vi "Vision Processing.vi"(4 "error in (no error)":errorcluster, 7 "Image Size":T4=enum."320x240") -> ()   [LabVIEW 2020]
doc: "This VI runs in parallel to other tasks. It gets images from the camera, processes them for color or shape and use that information to affect robot behavior."
uses:
  Robot Global Data.vi
  <vilib>/Rock Robotics/WPI/Camera/WPI_CameraWhite Balance Values.ctl
  <vilib>/Rock Robotics/WPI/Camera/WPI_CameraExposure Values.ctl
  <vilib>/Rock Robotics/WPI/Camera/WPI_CameraFrameRate.ctl
  <vilib>/Rock Robotics/Network Tables/NT Read Number.vi
  <vilib>/Rock Robotics/Network Tables/NT Write Boolean.vi
  <vilib>/Rock Robotics/Network Tables/NT Write Number.vi
  <vilib>/Rock Robotics/Network Tables/NT Read Boolean.vi
  <vilib>/Rock Robotics/WPI/Camera/WPI_CameraImageSize.ctl
panel:
  in  "Std Devs":cluster{"Hue":dbl, "Sat":dbl, "Val":dbl}={"Hue"=4.0, "Sat"=6.0, "Val"=4.0}
  in  "Color Components":T1={"Hue"={243.23333311080933, 20.233333110809326}, "Sat"={125.60287475585938, 242.93045043945312}, "Val"={83.88507843017578, 225.38158416748047}} {"Val" scale=0.0..255.0; "Sat" scale=0.0..255.0; "Hue" scale=0.0..255.0 scale format="%#_3g"}
  out "Fitted Mask":T2(plugin-control)
  in  "Targets":i32=3
  in  "Score Cutoff":dbl(slide)=70.58823529411765 scale=0.0..100.0
  out "Ranked Objects":T3(array[cluster]) {"Score" format="%#.1g"}
  in  "Annotations":enum16{"None", "Good", "All"}(ring)=enum."Good"
  in  "Area Size Limit %":dbl=0.4 format="%#_13g"
  out "Initial Mask":T2(plugin-control)
  out "Image":T2(plugin-control)
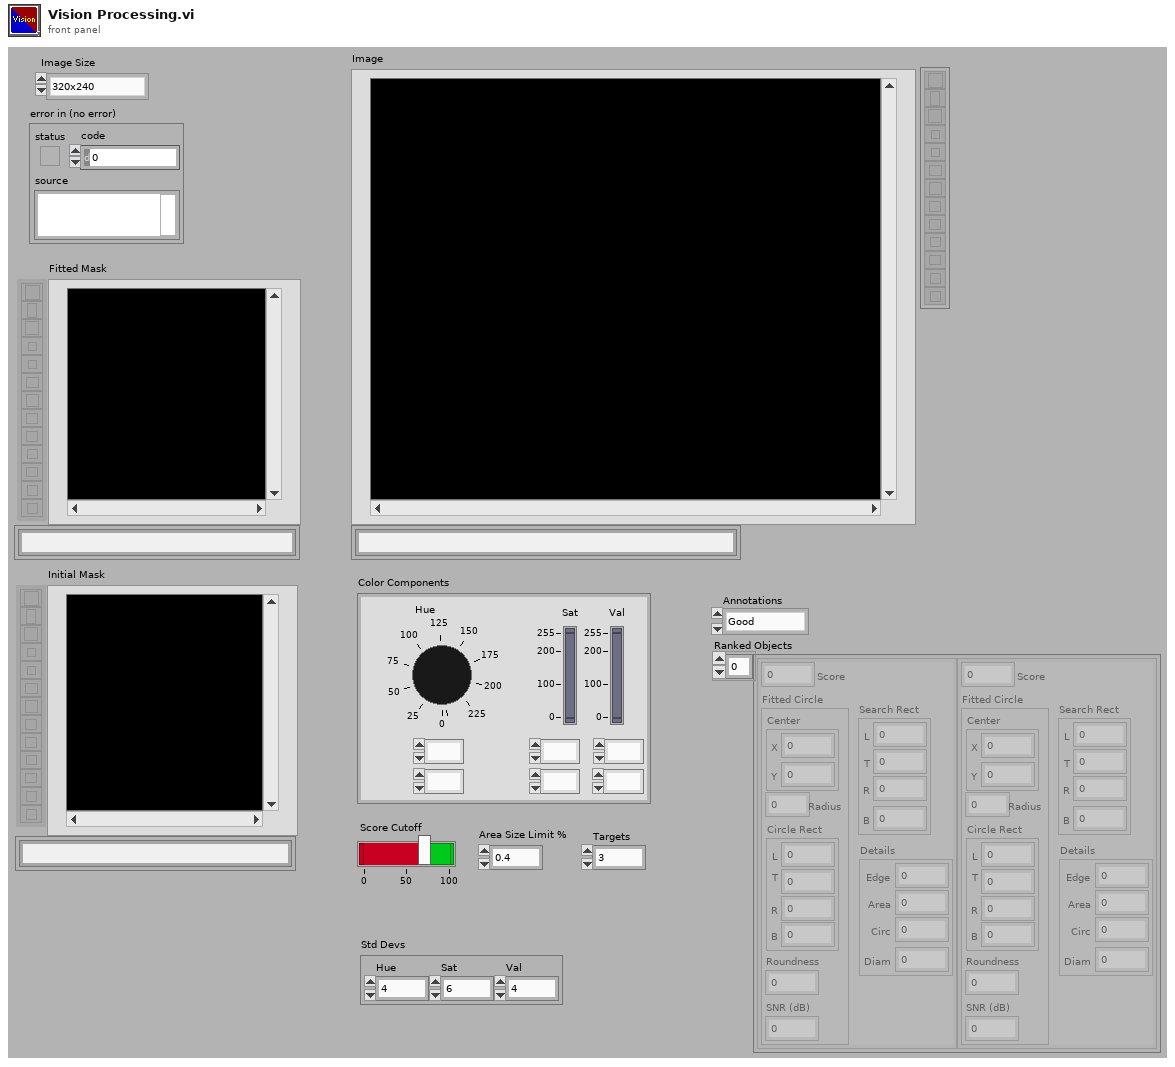
[diagram p1: front panel]
types:
  T1 = cluster{"Hue":cluster{dbl, dbl}, "Sat":cluster{dbl, dbl}, "Val":cluster{dbl, dbl}}
  T2 = typedef "IMAQ Image.ctl" = refnum<image>
  T3 = cluster{"Score":sgl, "Fitted Circle":cluster{"Center":cluster{"X":sgl, "Y":sgl}, "Radius":dbl, "Circle Rect":cluster{"L":sgl, "T":sgl, "R":sgl, "B":sgl}, "Roundness":dbl, "SNR (dB)":dbl}, "Search Rect":cluster{"L":sgl, "T":sgl, "R":sgl, "B":sgl}, "Details":cluster{"Edge":sgl, "Area":sgl, "Circ":sgl, "Diam":sgl}}[]
  T4 = typedef "WPI_CameraImageSize.ctl" = enum16{"640x480", "320x240", "160x120", "Custom"}
  T5 = typedef "WPI_CameraFrameRate.ctl" = u32
  T6 = typedef "WPI_CameraExposure Values.ctl" = enum16{"Auto", "Flicker-free 50 Hz", "Flicker-free 60 Hz", "Hold current", "Custom"}
  T7 = typedef "WPI_CameraWhite Balance Values.ctl" = enum16{"Auto", "Fixed indoor", "Fixed outdoor 1", "Fixed outdoor 2", "Fixed fluorescent 1", "Fixed fluorescent 2", "Hold current", "Custom"}
  T8 = typedef "Image Type" = u32
  T9 = typedef "WPI_CameraDevRef.ctl" = cluster{"Camera Address":string, "CameraStatus":errorcluster}
  T10 = typedef "WPI_DriverStationAllianceInfo.ctl" = enum16{"Red", "Blue", "Invalid"}
  T11 = cluster{cluster{"Numeric":dbl, "Numeric":dbl}, cluster{"Numeric":dbl, "Numeric":dbl}, cluster{"Numeric":dbl, "Numeric":dbl}}
  T12 = cluster{"Hue":cluster{"Numeric":dbl, "Numeric":dbl}, "Sat":cluster{"Numeric":dbl, "Numeric":dbl}, "Val":cluster{"Numeric":dbl, "Numeric":dbl}}
  T13 = cluster{"Circle Found":bool, "Fitted Circle":cluster{"Center":cluster{"X":sgl, "Y":sgl}, "Radius":dbl, "Center":cluster{"X":sgl, "Y":sgl}, "Radius":dbl, "Roundness":dbl, "Strength":dbl, "SNR (dB)":dbl}, "Array":dbl[], "Sorted Data":dbl[][]}[]
  T14 = cluster{cluster{dbl, dbl}, cluster{dbl, dbl}, cluster{dbl, dbl}}
  T15 = cluster{"Score":dbl, "Fitted Circle":cluster{"Center (Pixels)":cluster{"X":sgl, "Y":sgl}, "Radius (Pixels)":dbl, "Circle Rect":cluster{"Left":sgl, "Top":sgl, "Right":sgl, "Bottom":sgl}, "Roundness (RW)":dbl, "Average SNR (dB)":dbl}, "Search Rect":cluster{"Left":sgl, "Top":sgl, "Right":sgl, "Bottom":sgl}, "Details":cluster{"Edges":sgl, "Circ/Rect":sgl, "Diam/Diam":sgl, "Circularity":sgl}}[]
  T16 = cluster{"Object Info[0]":cluster{"Score":dbl, "Fitted Circle":cluster{"Center (Pixels)":cluster{"X":sgl, "Y":sgl}, "Radius (Pixels)":dbl, "Circle Rect":cluster{"Left":sgl, "Top":sgl, "Right":sgl, "Bottom":sgl}, "Roundness (RW)":dbl, "Average SNR (dB)":dbl}, "Search Rect":cluster{"Left":sgl, "Top":sgl, "Right":sgl, "Bottom":sgl}, "Details":cluster{"Edges":sgl, "Circ/Rect":sgl, "Diam/Diam":sgl, "Circularity":sgl}}, "Object Info[1]":cluster{"Score":dbl, "Fitted Circle":cluster{"Center (Pixels)":cluster{"X":sgl, "Y":sgl}, "Radius (Pixels)":dbl, "Circle Rect":cluster{"Left":sgl, "Top":sgl, "Right":sgl, "Bottom":sgl}, "Roundness (RW)":dbl, "Average SNR (dB)":dbl}, "Search Rect":cluster{"Left":sgl, "Top":sgl, "Right":sgl, "Bottom":sgl}, "Details":cluster{"Edges":sgl, "Circ/Rect":sgl, "Diam/Diam":sgl, "Circularity":sgl}}, "Object Info[2]":cluster{"Score":dbl, "Fitted Circle":cluster{"Center (Pixels)":cluster{"X":sgl, "Y":sgl}, "Radius (Pixels)":dbl, "Circle Rect":cluster{"Left":sgl, "Top":sgl, "Right":sgl, "Bottom":sgl}, "Roundness (RW)":dbl, "Average SNR (dB)":dbl}, "Search Rect":cluster{"Left":sgl, "Top":sgl, "Right":sgl, "Bottom":sgl}, "Details":cluster{"Edges":sgl, "Circ/Rect":sgl, "Diam/Diam":sgl, "Circularity":sgl}}, "Object Info[3]":cluster{"Score":dbl, "Fitted Circle":cluster{"Center (Pixels)":cluster{"X":sgl, "Y":sgl}, "Radius (Pixels)":dbl, "Circle Rect":cluster{"Left":sgl, "Top":sgl, "Right":sgl, "Bottom":sgl}, "Roundness (RW)":dbl, "Average SNR (dB)":dbl}, "Search Rect":cluster{"Left":sgl, "Top":sgl, "Right":sgl, "Bottom":sgl}, "Details":cluster{"Edges":sgl, "Circ/Rect":sgl, "Diam/Diam":sgl, "Circularity":sgl}}, "Object Info[4]":cluster{"Score":dbl, "Fitted Circle":cluster{"Center (Pixels)":cluster{"X":sgl, "Y":sgl}, "Radius (Pixels)":dbl, "Circle Rect":cluster{"Left":sgl, "Top":sgl, "Right":sgl, "Bottom":sgl}, "Roundness (RW)":dbl, "Average SNR (dB)":dbl}, "Search Rect":cluster{"Left":sgl, "Top":sgl, "Right":sgl, "Bottom":sgl}, "Details":cluster{"Edges":sgl, "Circ/Rect":sgl, "Diam/Diam":sgl, "Circularity":sgl}}, "Object Info[5]":cluster{"Score":dbl, "Fitted Circle":cluster{"Center (Pixels)":cluster{"X":sgl, "Y":sgl}, "Radius (Pixels)":dbl, "Circle Rect":cluster{"Left":sgl, "Top":sgl, "Right":sgl, "Bottom":sgl}, "Roundness (RW)":dbl, "Average SNR (dB)":dbl}, "Search Rect":cluster{"Left":sgl, "Top":sgl, "Right":sgl, "Bottom":sgl}, "Details":cluster{"Edges":sgl, "Circ/Rect":sgl, "Diam/Diam":sgl, "Circularity":sgl}}, "Object Info[6]":cluster{"Score":dbl, "Fitted Circle":cluster{"Center (Pixels)":cluster{"X":sgl, "Y":sgl}, "Radius (Pixels)":dbl, "Circle Rect":cluster{"Left":sgl, "Top":sgl, "Right":sgl, "Bottom":sgl}, "Roundness (RW)":dbl, "Average SNR (dB)":dbl}, "Search Rect":cluster{"Left":sgl, "Top":sgl, "Right":sgl, "Bottom":sgl}, "Details":cluster{"Edges":sgl, "Circ/Rect":sgl, "Diam/Diam":sgl, "Circularity":sgl}}, "Object Info[7]":cluster{"Score":dbl, "Fitted Circle":cluster{"Center (Pixels)":cluster{"X":sgl, "Y":sgl}, "Radius (Pixels)":dbl, "Circle Rect":cluster{"Left":sgl, "Top":sgl, "Right":sgl, "Bottom":sgl}, "Roundness (RW)":dbl, "Average SNR (dB)":dbl}, "Search Rect":cluster{"Left":sgl, "Top":sgl, "Right":sgl, "Bottom":sgl}, "Details":cluster{"Edges":sgl, "Circ/Rect":sgl, "Diam/Diam":sgl, "Circularity":sgl}}, "Object Info[8]":cluster{"Score":dbl, "Fitted Circle":cluster{"Center (Pixels)":cluster{"X":sgl, "Y":sgl}, "Radius (Pixels)":dbl, "Circle Rect":cluster{"Left":sgl, "Top":sgl, "Right":sgl, "Bottom":sgl}, "Roundness (RW)":dbl, "Average SNR (dB)":dbl}, "Search Rect":cluster{"Left":sgl, "Top":sgl, "Right":sgl, "Bottom":sgl}, "Details":cluster{"Edges":sgl, "Circ/Rect":sgl, "Diam/Diam":sgl, "Circularity":sgl}}}
  T17 = cluster{"Score":dbl, "Fitted Circle":cluster{"Center (Pixels)":cluster{"X":sgl, "Y":sgl}, "Radius (Pixels)":dbl, "Circle Rect":cluster{"Left":sgl, "Top":sgl, "Right":sgl, "Bottom":sgl}, "Roundness (RW)":dbl, "Average SNR (dB)":dbl}, "Search Rect":cluster{"Left":sgl, "Top":sgl, "Right":sgl, "Bottom":sgl}, "Details":cluster{"Edges":sgl, "Circ/Rect":sgl, "Diam/Diam":sgl, "Circularity":sgl}}
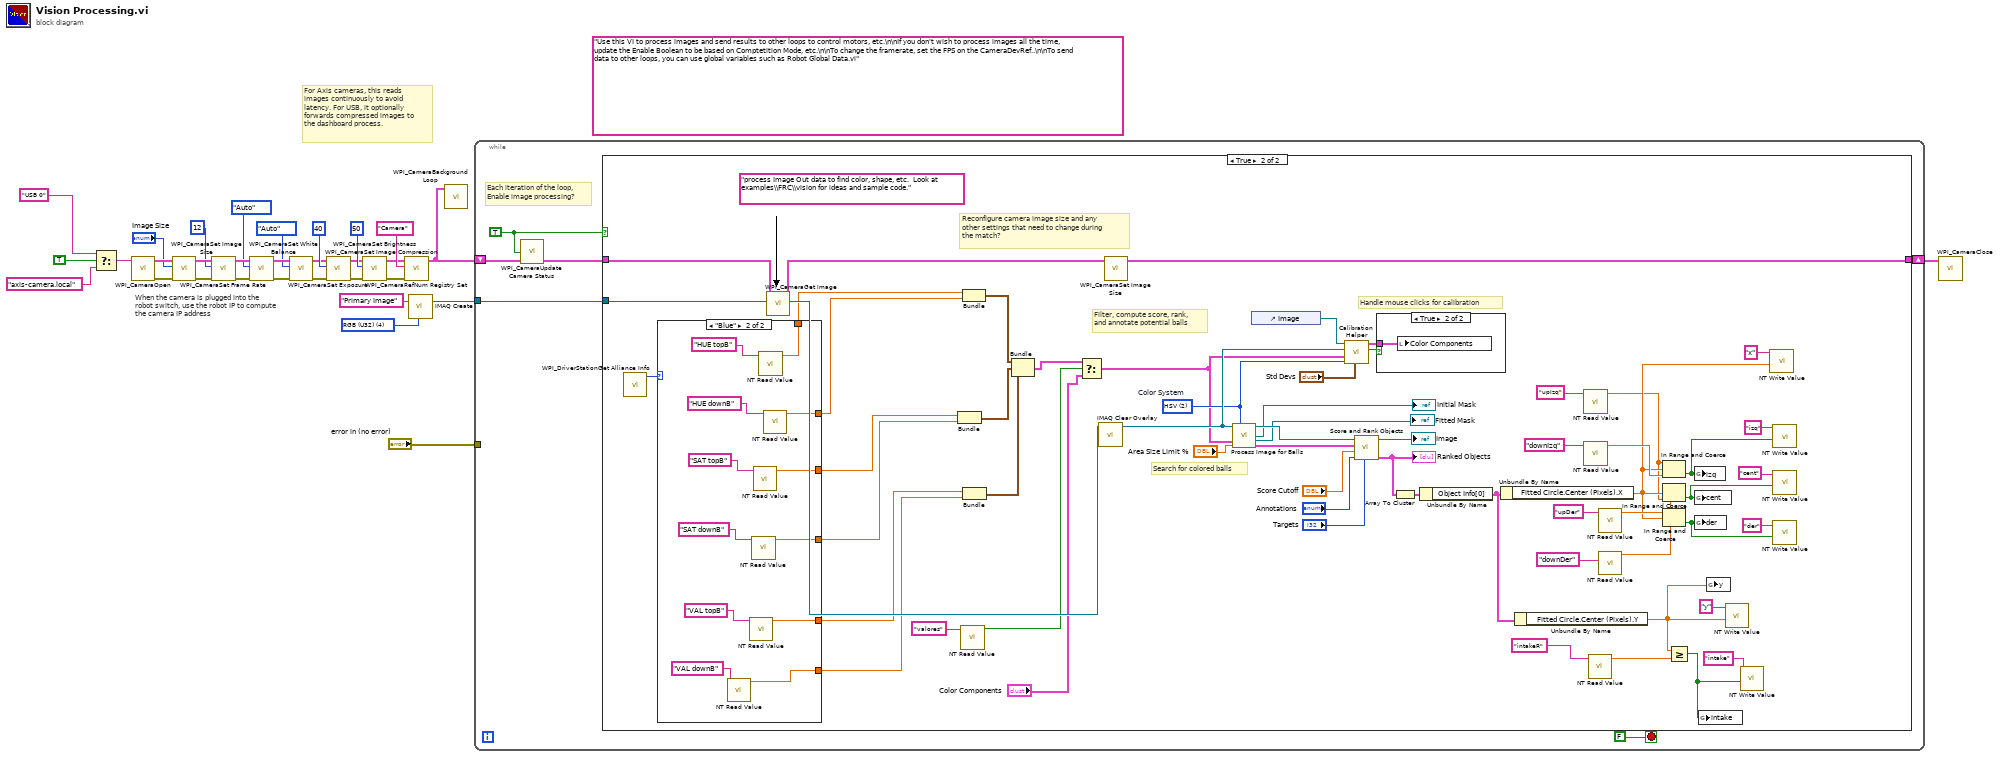
[diagram p0: block diagram]
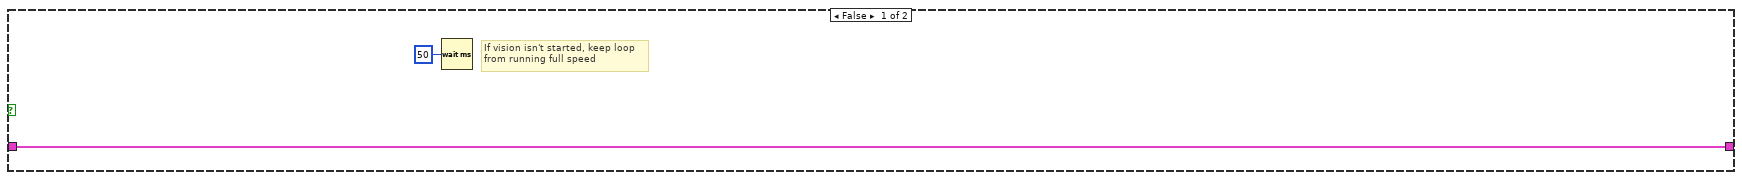
[diagram p2: hidden frame]
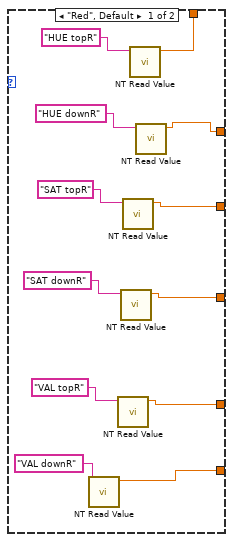
[diagram p3: hidden frame]
diagram:
  (unwired) "Use this VI to process images and send results to other loops to control motors, etc.\n\nIf you don't wish to process images all the time, update the Enable Boolean to be based on Comptetition Mode, etc.\n\nTo change the framerate, set the FPS on the CameraDevRef..\n\nTo send data to other loops, you can use global variables such as Robot Global Data.vi"
  w31 = T8 4 items=["Grayscale (U8)", "Grayscale (I16)", "Grayscale (SGL)", "Complex (CSG)", "RGB (U32)", "HSL (U32)", "RGB (U64)"] ("Image Type")
  # "When the camera is plugged into the\nrobot switch, use the robot IP to compute\nthe camera IP address"
  # "For Axis cameras, this reads\nimages continuously to avoid\nlatency. For USB, it optionally\nforwards compressed images to\nthe dashboard process."
  n1 = Select(t="USB 0", s=TRUE ("dot notation? (F)"), f="axis-camera.local" ("format string")) -> (s? t:f=w3:string)
  n2 = call <vilib>:"WPI_CameraOpen.vi"("Camera Address"=w3) -> ("error out"=w19:errorcluster, "CameraDevRef"=w20:T9)  [unwired: 2 in, 7 out]
  n3 = call <vilib>:"WPI_CameraSet Image Size.vi"("error in (no error)"=w19, "Image Size"="Image Size", "CameraDevRef"=w20) -> ("error out"=w18:errorcluster, "CameraDevRef Out"=w21:T9)  [unwired: 1 in, 6 out]
  n4 = call <vilib>:"WPI_CameraSet Frame Rate.vi"("error in (no error)"=w18, "Frame Rate (fps)"=T5 12, "CameraDevRef"=w21) -> ("error out"=w17:errorcluster, "CameraDevRef Out"=w23:T9)  [unwired: 7 out]
  n5 = call <vilib>:"WPI_CameraSet White Balance.vi"("error in (no error)"=w17, "White Balance"=WPI_CameraWhite_Balance_Values."Auto", "CameraDevRef"=w23) -> ("error out"=w16:errorcluster, "CameraDevRef Out"=w22:T9)  [unwired: 1 in, 6 out]
  n6 = call <vilib>:"WPI_CameraSet Exposure.vi"("error in (no error)"=w16, "Exposure"=WPI_CameraExposure_Values."Auto", "CameraDevRef"=w22) -> ("error out"=w15:errorcluster, "CameraDevRef Out"=w25:T9)  [unwired: 1 in, 6 out]
  n7 = call <vilib>:"WPI_CameraSet Image Compression.vi"("error in (no error)"=w15, "Compression"=40, "CameraDevRef"=w25) -> ("error out"=w14:errorcluster, "CameraDevRef Out"=w24:T9)  [unwired: 7 out]
  n8 = call <vilib>:"WPI_CameraSet Brightness.vi"("error in (no error)"=w14, "Brightness"=50, "CameraDevRef"=w24) -> ("error out"=w12:errorcluster, "CameraDevRef Out"=w13:T9)  [unwired: 1 in, 6 out]
  n9 = call <vilib>:"WPI_CameraRefNum Registry Set.vi"("error in (no error)"=w12, "refnum name"="Camera", "CameraDevRef"=w13) -> ("CameraDevRef"=w8:T9)  [unwired: 1 in, 7 out]
  n10 = call "IMAQ Create"("Image Name"="Primary Image", "Image Type"=w31) -> ("New Image"=w29:T2)  [unwired: 2 in, 2 out]
  n11 = call <vilib>:"WPI_CameraBackground Loop.vi"("CameraDevRef"=w8) -> ()  [unwired: 11 in]
  n12 = while {
    shift-right: [w36] -> w6
    shift-left: w8 -> [w34]
    tunnel: w29 -> [w35]
    tunnel: "error in (no error)" -> [_]
    stop <- FALSE stop-if-true
    w32 = TRUE
    # "Each iteration of the loop,\nEnable image processing?"
    n13 = call <vilib>:"WPI_CameraUpdate Camera Status.vi"("CameraDevRef In"=w34, "Enable Vision"=w32) -> ("CameraDevRef Out"=w33:T9)  [unwired: 3 in]
    n14 = case shown="True" w32 {
      tunnel: w35 -> [_ w96]
      tunnel: [w39 w99] -> w36
      tunnel: w33 -> [w39 w98]
      frame False {
        # "If vision isn't started, keep loop\nfrom running full speed"
        n15 = Wait (ms)(milliseconds to wait=u32 50) -> ()  [unwired: 1 out]
      }
      frame True {
        w85 = u16 2 items=["RGB", "HSL", "HSV", "HSI"]  # Color System
        (unwired) "process Image Out data to find color, shape, etc.  Look at examples\\FRC\\vision for ideas and sample code."
        # "Handle mouse clicks for calibration"
        # "Search for colored balls"
        # "Filter, compute score, rank,\nand annotate potential balls"
        # "Reconfigure camera image size and any\nother settings that need to change during\nthe match?"
        n16 = call <vilib>:"WPI_DriverStationGet Alliance Info.vi"() -> ("Alliance"=w46:T10)  [unwired: 6 in, 5 out]
        n17 = case shown="\"Blue\"" w46 {
          tunnel: [w100 w117] -> w45
          tunnel: [w103 w116] -> w44
          tunnel: [w101 w115] -> w43
          tunnel: [w102 w114] -> w42
          tunnel: [w104 w113] -> w41
          tunnel: [w105 w112] -> w40
          frame "Red", Default {
            n18 = call-poly <vilib>:"NT Read Value.vi"("Name"="VAL downR") -> ("Numeric"=w100:dbl)  [unwired: 9 in, 1 out]
            n19 = call-poly <vilib>:"NT Read Value.vi"("Name"="VAL topR") -> ("Numeric"=w101:dbl)  [unwired: 9 in, 1 out]
            n20 = call-poly <vilib>:"NT Read Value.vi"("Name"="SAT downR") -> ("Numeric"=w102:dbl)  [unwired: 9 in, 1 out]
            n21 = call-poly <vilib>:"NT Read Value.vi"("Name"="SAT topR") -> ("Numeric"=w103:dbl)  [unwired: 9 in, 1 out]
            n22 = call-poly <vilib>:"NT Read Value.vi"("Name"="HUE topR") -> ("Numeric"=w105:dbl)  [unwired: 9 in, 1 out]
            n23 = call-poly <vilib>:"NT Read Value.vi"("Name"="HUE downR") -> ("Numeric"=w104:dbl)  [unwired: 9 in, 1 out]
          }
          frame "Blue" {
            n24 = call-poly <vilib>:"NT Read Value.vi"("Name"="VAL downB") -> ("Numeric"=w117:dbl)  [unwired: 9 in, 1 out]
            n25 = call-poly <vilib>:"NT Read Value.vi"("Name"="VAL topB") -> ("Numeric"=w115:dbl)  [unwired: 9 in, 1 out]
            n26 = call-poly <vilib>:"NT Read Value.vi"("Name"="SAT downB") -> ("Numeric"=w114:dbl)  [unwired: 9 in, 1 out]
            n27 = call-poly <vilib>:"NT Read Value.vi"("Name"="SAT topB") -> ("Numeric"=w116:dbl)  [unwired: 9 in, 1 out]
            n28 = call-poly <vilib>:"NT Read Value.vi"("Name"="HUE topB") -> ("Numeric"=w112:dbl)  [unwired: 9 in, 1 out]
            n29 = call-poly <vilib>:"NT Read Value.vi"("Name"="HUE downB") -> ("Numeric"=w113:dbl)  [unwired: 9 in, 1 out]
          }
        }
        n30 = call <vilib>:"WPI_CameraGet Image.vi"("Image"=w96, "CameraDevRef"=w98) -> ("Image Out"=w62:T2, "CameraDevRef Out"=w97:T9)  [unwired: 1 in, 7 out]
        n31 = Bundle("Numeric"=w44, "Numeric"=w42) -> (w60:cluster{"Numeric":dbl, "Numeric":dbl})  [unwired: 1 in]
        n32 = call-poly <vilib>:"NT Read Value.vi"("Name"="valores") -> ("Boolean"=w54:bool)  [unwired: 9 in, 1 out]
        n33 = Bundle("Numeric"=w40, "Numeric"=w41) -> (w61:cluster{"Numeric":dbl, "Numeric":dbl})  [unwired: 1 in]
        n34 = Bundle("Numeric"=w43, "Numeric"=w45) -> (w59:cluster{"Numeric":dbl, "Numeric":dbl})  [unwired: 1 in]
        n35 = Bundle(w61, w60, w59) -> (w55:T11)  [unwired: 1 in]
        n36 = Select(t=w55, s=w54, f="Color Components") -> (s? t:f=w56:T12)
        n37 = call "IMAQ Clear Overlay"("Image"=w62) -> ("Image Out"=w92:T2)  [unwired: 9 in, 1 out]
        n38 = call <vilib>:"WPI_CameraSet Image Size.vi"("CameraDevRef"=w97) -> ("CameraDevRef Out"=w99:T9)  [unwired: 3 in, 7 out]
        n39 = call "Process Image for Balls.vi"("Src Image"=w92, "Color Mode 2"=w85, "Color"=w56, "Area Cutoff %"="Area Size Limit %") -> ("Src Image Out"=w90:T2, "First Threshold"=→"Initial Mask":T2, "Fitted"=→"Fitted Mask":T2, "Potential"=w89:T13)  [unwired: 8 in]
        n40 = control-ref of="Image"() -> (w84:refnum<vi>)
        n41 = call "Calibration Helper.vi"("Std Devs"="Std Devs", "Color Mode"=w85, "Color Components"=w56, "Image"=w92, "Image Ctl Refnum"=w84) -> ("Changed"=w81:bool, "output color"=w83:T14)  [unwired: 5 in]
        n42 = call "Score and Rank Objects.vi"("Targets"="Targets", "Annotations"="Annotations", "Score Limit"="Score Cutoff", "Object Info"=w89, "Image in"=w90) -> ("Object Info"=w80:T15, "Annotated Image"=→"Image":T2)  [unwired: 5 in]
        "Ranked Objects" <- w80
        n43 = case shown="True" w81 {
          tunnel: w83 -> [_ w124]
          frame False {
          }
          frame True {
            n44 = local write "Color Components"(w124) -> ()
          }
        }
        n45 = Array To Cluster(array=w80) -> (cluster=w79:T16)
        n46 = Unbundle By Name(w79) -> ("Object Info[0]"=w52:T17)
        n47 = Unbundle By Name(w52) -> ("Fitted Circle.Center (Pixels).X"=w66:sgl)
        n48 = Unbundle By Name(w52) -> ("Fitted Circle.Center (Pixels).Y"=w48:sgl)
        n49 = call-poly <vilib>:"NT Read Value.vi"("Name"="upIzq") -> ("Numeric"=w63:dbl)  [unwired: 9 in, 1 out]
        n50 = call-poly <vilib>:"NT Read Value.vi"("Name"="downIzq") -> ("Numeric"=w77:dbl)  [unwired: 9 in, 1 out]
        n51 = call-poly <vilib>:"NT Read Value.vi"("Name"="intakeR") -> ("Numeric"=w50:dbl)  [unwired: 9 in, 1 out]
        n52 = call-poly <vilib>:"NT Read Value.vi"("Name"="upDer") -> ("Numeric"=w78:dbl)  [unwired: 9 in, 1 out]
        n53 = call-poly <vilib>:"NT Read Value.vi"("Name"="downDer") -> ("Numeric"=w64:dbl)  [unwired: 9 in, 1 out]
        n54 = In Range and Coerce(upper limit=w63, x=w66, lower limit=w77) -> (In Range?=w70:bool)  [unwired: 1 out]
        n55 = In Range and Coerce(upper limit=w64, x=w66, lower limit=w63) -> (In Range?=w71:bool)  [unwired: 1 out]
        n56 = In Range and Coerce(upper limit=w78, x=w66, lower limit=w64) -> (In Range?=w72:bool)  [unwired: 1 out]
        n57 = Greater Or Equal?(x=w48, y=w50) -> (x >= y?=w47:bool)
        n58 = global write "Robot Global Data.vi" "izq"(w70) -> ()
        n59 = global write "Robot Global Data.vi" "cent"(w71) -> ()
        n60 = global write "Robot Global Data.vi" "der"(w72) -> ()
        n61 = global write "Robot Global Data.vi" "intake"(w47) -> ()
        n62 = global write "Robot Global Data.vi" "y"(w48) -> ()
        n63 = call-poly <vilib>:"NT Write Value.vi"("Numeric"=w48, "Name"="y") -> ()  [unwired: 9 in, 1 out]
        n64 = call-poly <vilib>:"NT Write Value.vi"("Boolean"=w47, "Name"="intake") -> ()  [unwired: 9 in, 1 out]
        n65 = call-poly <vilib>:"NT Write Value.vi"("Numeric"=w66, "Name"="x") -> ()  [unwired: 9 in, 1 out]
        n66 = call-poly <vilib>:"NT Write Value.vi"("Boolean"=w70, "Name"="izq") -> ()  [unwired: 9 in, 1 out]
        n67 = call-poly <vilib>:"NT Write Value.vi"("Boolean"=w71, "Name"="cent") -> ()  [unwired: 9 in, 1 out]
        n68 = call-poly <vilib>:"NT Write Value.vi"("Boolean"=w72, "Name"="der") -> ()  [unwired: 9 in, 1 out]
      }
    }
  }
  n69 = call <vilib>:"WPI_CameraClose.vi"("CameraDevRef"=w6) -> ()  [unwired: 1 in, 10 out]
